vi "Global_OnCommand.vi"(10 "Command ID":string, 11 "Object":T1) -> ()   [LabVIEW 2020, in "FlexWorker_Provider.lvlib"]
uses:
  FlexWorker_Provider.lvlib
  <resource>/Framework/Providers/API/ItemRef.ctl
  FlexBlocks/FlexBlocks.lvlib
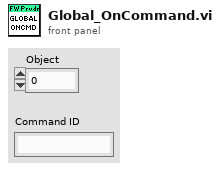
[diagram p1: front panel]
types:
  T1 = typedef "ItemRef.ctl" = u64
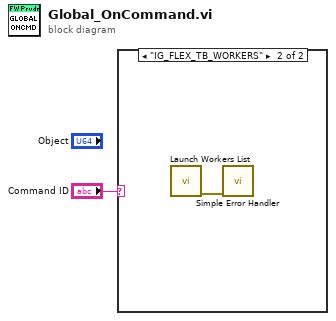
[diagram p0: block diagram]
diagram:
  n1 = case shown="\"IG_FLEX_TB_WORKERS\"" "Command ID" {
    frame "False", Default {
    }
    frame "IG_FLEX_TB_WORKERS" {
      n2 = call "Launch Workers List.vi"() -> ("error out"=w2:errorcluster)  [unwired: 11 in]
      n3 = call <vilib>:"Simple Error Handler.vi"("error in (no error)"=w2) -> ()  [unwired: 4 in, 5 out]
    }
  }
